vi "Untitled 3.vi"() -> ()   [LabVIEW 2017]
panel:
  out "indicator=1 if a+b>a*b":bool
  out "a/b":dbl
  out "a*b":dbl
  out "a_b":dbl
  out "a+b":dbl
  in  "b":dbl
  in  "a":dbl
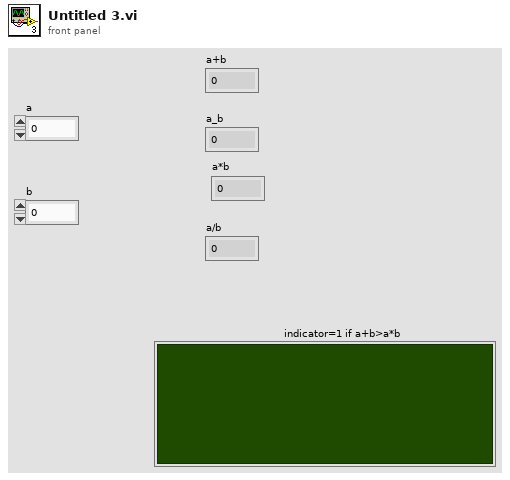
[diagram p1: front panel]
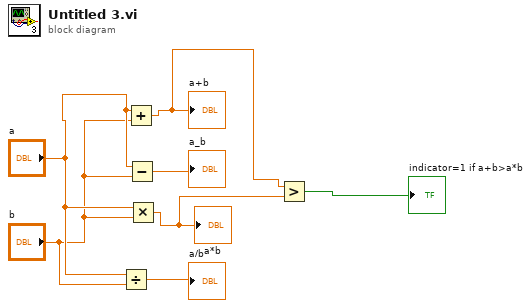
[diagram p0: block diagram]
diagram:
  n1 = Divide(x="a", y="b") -> (x/y=→"a/b":dbl)
  n2 = Add(x="a", y="b") -> (x+y=w2:dbl)
  "a+b" <- w2
  n3 = Subtract(x="a", y="b") -> (x-y=→"a_b":dbl)
  n4 = Multiply(x="a", y="b") -> (x*y=w1:dbl)
  "a*b" <- w1
  n5 = Greater?(x=w2, y=w1) -> (0:→"indicator=1 if a+b>a*b":bool)
